vi "The End of the RUN.vi"(8 "error in (no error)":errorcluster, 11 "Monkey in":refnum<class "Monkey.lvclass">) -> (0 "error out":errorcluster, 3 "Monkey out":refnum<class "Monkey.lvclass">)   [LabVIEW 2020, in "Monkey.lvlib" / "Monkey.lvclass"]
doc: "VI called after each Run Finishes correctly. It removes Current Run and appends it to the schedule if the continuous flag is on."
uses:
  Monkey.lvclass
  Monkey.lvclass/Monkey.ctl
  Run Utilities/Run Instance/Run Instance.lvclass
  Ancestor/Ancestor/Ancestor.lvclass/Ancestor.ctl
  Support VIs/Generate Error.vi
  FGV/Error Memory/Get Error Description.vi
  Support VIs/Get PC name.vi
  Ancestor/Ancestor/Read ID.vi
  Support VIs/Get Class Name.vi
  <vilib>/Utility/error.llb/Clear Errors.vi
  FGV/Error Memory/Error Memory Core.vi
  <vilib>/AdvancedString/Delimited String to 1D String Array.vi
  Support VIs/Circus Root Path.vi
  FGV/Error Memory/Error Crt Lvl checker.vi
  FGV/Error Memory/Error Memory Core.vi/40c8088d-b597-4017-91af-faa98e00292e.vi
  FGV/Error Memory/Error Memory Core.vi/d4a3ab98-063c-4e44-b43d-fbdcfe6c2be2.vi
  Support VIs/Global Memory.vi
  <vilib>/Utility/LVClass/Get LV Class Name.vi
  Support VIs/Is in Packed Library.vi
  Support VIs/TALOS Root path.vi
  Support VIs/Read CSV worksheet.vi
  Support VIs/Global Constants.vi
  <vilib>/Utility/error.llb/General Error Handler.vi
  Support VIs/Error Log.vi
  Run Utilities/Schedule/Schedule.lvclass
  Ancestor/Ancestor/Ancestor.lvclass
  <vilib>/Comparison/Equal/Equal Functor/Equal Functor.lvclass
  Run Utilities/Run Block/Run Block.lvclass
  Run Utilities/Cell/Schedule Cell.lvclass
  TALOS.lvlib
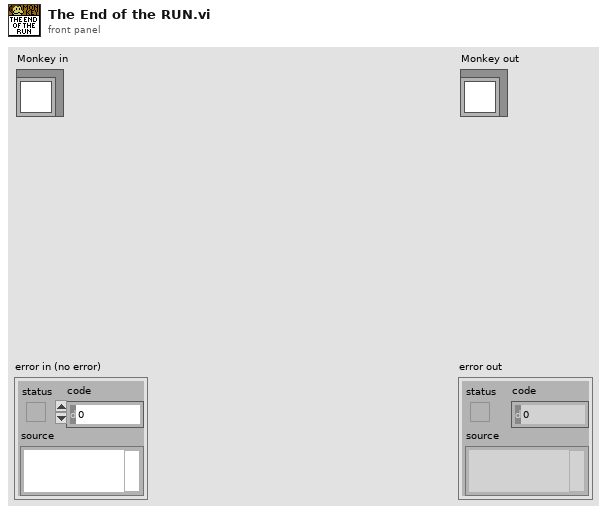
[diagram p1: front panel]
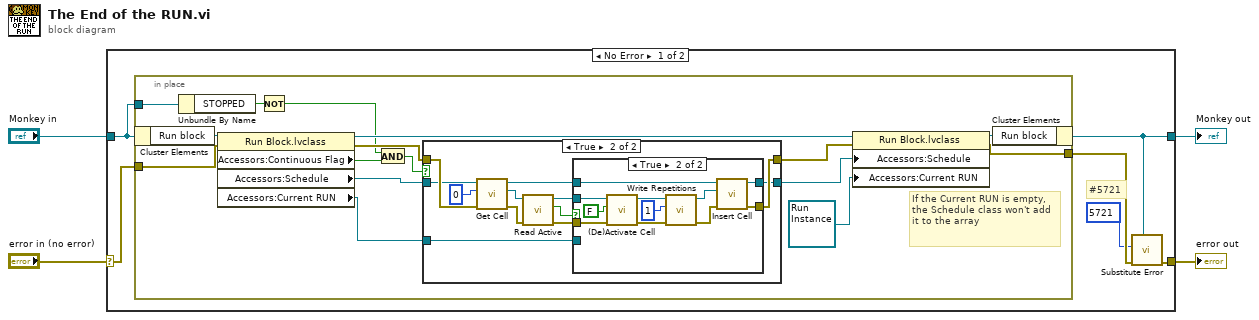
[diagram p0: block diagram]
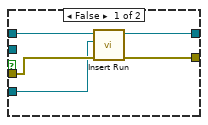
[diagram p3: hidden frame]
diagram:
  n1 = case shown="No Error" "error in (no error)" {
    selector: "error in (no error)" -> [w10 w58]
    tunnel: [w9 w58] -> w3
    tunnel: [w7 w57] -> w1
    tunnel: "Monkey in" -> [w5 w57]
    frame No Error {
      # "#5721"
      n2 = in-place {
        in-place-border: w10 -> [w18]
        in-place-border: [w25] -> w8
        in-place-border: w5 -> [w13]
        # "If the Current RUN is empty, the Schedule class won't add it to the array"
        n3 = in-place-cluster #1(w5) -> ("Run block"=w19:refnum<class "Run Block.lvclass">)
        n4 = Unbundle By Name(w13) -> ("STOPPED"=w12:bool)
        n5 = property class="Run Block.lvclass"(reference=w19, error in=w18) -> (reference out=w24:refnum<class "Run Block.lvclass">, error out=w17:errorcluster, "Accessors:Continuous Flag"=w14:bool, "Accessors:Schedule"=w23:refnum<class "Schedule.lvclass">, "Accessors:Current RUN"=w22:refnum<class "Run Instance.lvclass">)
        n6 = Not(x=w12) -> (.not. x?=w11:bool)
        n7 = And(x=w11, y=w14) -> (x .and. y?=w15:bool)
        n8 = case shown="True" w15 {
          tunnel: w17 -> [w28 w39]
          tunnel: w23 -> [w27 w38]
          tunnel: w22 -> [_ w30]
          tunnel: [w28 w40] -> w21
          tunnel: [w27 w31] -> w20
          frame False {
          }
          frame True {
            n9 = call-dynamic "Get Cell.vi"("error in (no error)"=w39, "index"=0, "Schedule in"=w38) -> ("error out"=w36:errorcluster, "Schedule Cell"=w37:refnum<class "Schedule Cell.lvclass">, "Schedule out"=w32:refnum<class "Schedule.lvclass">)  [unwired: 6 in]
            n10 = call-dynamic "Read Active.vi"("error in (no error)"=w36, "Schedule Cell in"=w37) -> ("error out"=w34:errorcluster, "Active"=w33:bool, "Schedule Cell out"=w35:refnum<class "Schedule Cell.lvclass">)  [unwired: 7 in]
            n11 = case shown="True" w33 {
              tunnel: w35 -> [_ w50]
              tunnel: w34 -> [w43 w48]
              tunnel: w32 -> [w45 w55]
              tunnel: [w44 w54] -> w31
              tunnel: w30 -> [w42 _]
              tunnel: [w41 w53] -> w40
              frame False {
                n12 = call-dynamic "Insert Run.vi"("error in (no error)"=w43, "Run Instance"=w42, "Schedule in"=w45) -> ("error out"=w41:errorcluster, "Schedule out"=w44:refnum<class "Schedule.lvclass">)  [unwired: 6 in, 1 out]
              }
              frame True {
                n13 = call-dynamic "(De)Activate Cell.vi"("error in (no error)"=w48, "Active"=FALSE, "Schedule Cell in"=w50) -> ("error out"=w47:errorcluster, "Schedule Cell out"=w49:refnum<class "Schedule Cell.lvclass">)  [unwired: 7 in]
                n14 = call-dynamic "Write Repetitions.vi"("error in (no error)"=w47, "Repetitions"=u32 1, "Schedule Cell in"=w49) -> ("error out"=w52:errorcluster, "Schedule Cell out"=w51:refnum<class "Schedule Cell.lvclass">)  [unwired: 7 in]
                n15 = call-dynamic "Insert Cell.vi"("error in (no error)"=w52, "Schedule Cell"=w51, "Schedule in"=w55) -> ("error out"=w53:errorcluster, "Schedule out"=w54:refnum<class "Schedule.lvclass">)  [unwired: 7 in]
              }
            }
          }
        }
        n16 = property class="Run Block.lvclass"(reference=w24, error in=w21, "Accessors:Schedule"=w20, "Accessors:Current RUN"=refnum<class "Run Instance.lvclass"> refnum ("Current RUN")) -> (reference out=w26:refnum<class "Run Block.lvclass">, error out=w25:errorcluster)
        n17 = in-place-cluster #1("Run block"=w26) -> (w7:refnum<class "Monkey.lvclass">)
      }
      n18 = call "Substitute Error.vi"("LabVIEW Object"=w7, "error in (no error)"=w8, "Error Code"=5721) -> ("error out"=w9:errorcluster)  [unwired: 8 in]
    }
    frame Error {
    }
  }
  "error out" <- w3
  "Monkey out" <- w1
